vi "Vision Processing.vi"(4 "error in (no error)":errorcluster, 6 "CameraDevRef":T1) -> ()   [LabVIEW 2011]
uses:
  <vilib>/Rock Robotics/WPI/Camera/WPI_CameraDevRef.ctl
  Robot Global Data.vi
  <vilib>/vision/NI_Vision_Development_Module.lvlib
panel:
  in  "Scale":bool=TRUE
  out "Waveform Chart":dynamicdata(graph)
  out "Turret Movement Time":u32
  out "Target Identify Time":u32
  in  "Run Calculations":bool
  out "Raw Turret":dbl
  out "Target X Coord":dbl
  out "Target Distance":dbl
  out "Target Y Coord":dbl
  out "Distance Array":dbl[](array[numeric])
  in  "Scaler":dbl=0.85
  in  "Lower Speed Limit":dbl=0.05
  out "Number of Rectangles Visible":dbl
  out "Y Position Array":dbl[](array[numeric])
  out "X Position Array":dbl[](array[numeric])
  in  "View":bool
  out "Target Info":T2(array[cluster])
  in  "Area Size Limit":i32=444
  in  "Particle Count Limit":i32=8
  in  "Score Limits":T3={"Rect Coverage"=76.0, "Aspect Ratio"=40.0, "X Edge Strength"=40.0, "Y Edge Strength"=60.0}
  in  "Processing":enum32{"Color", "Intensity", "Intensity Open"}(tab)=enum."Intensity Open"
  in  "Luminance":i32=255
  in  "Saturation":i32=255
  in  "Hue":i32(knob)=65 scale=0.0..255.0
  in  "Margins":cluster{"Hue":i32, "Sat":i32, "Lum":i32}={"Hue"=20, "Sat"=27, "Lum"=30} {"Sat" scale=0.0..40.0; "Lum" scale=0.0..40.0; "Hue" scale=0.0..40.0}
  in  "Range":cluster{"Lower value":sgl, "Upper value":sgl}={"Lower value"=150.0, "Upper value"=255.0} {"Lower value" scale=0.0..255.0; "Upper value" scale=0.0..255.0}
  in  "Range":cluster{"Lower value":sgl, "Upper value":sgl}={"Lower value"=123.804344, "Upper value"=255.0} {"Lower value" scale=0.0..255.0; "Upper value" scale=0.0..255.0}
  in  "View":bool
  out "Processed Image":T4(plugin-control)
  out "Original Image":T4(plugin-control)
  # "Instructions:\nProcessing the reflective tape that is illuminated by a ring light can be based\non color or light intensity.\nParticles within the image are scored by rectangle coverage, aspect ratio, and\nfor being hollow with a bold edge. A particle is considered a target if all scores\nare above the score limits. Particles can be annotated -- surrounded by\na rectangle and scores drawn to the left .\nTo control the number of particles being scored, use the count limit and the size\nlimit."
  # "No Scale"
  # "To debug, Enable using the View button.\nFor color processing, you can click in the image to select the color for processing."
  # "Enable by clicking the View button.\nGreen scores are above the limit, orange are below. Inner/outer rect\nindicates all passed."
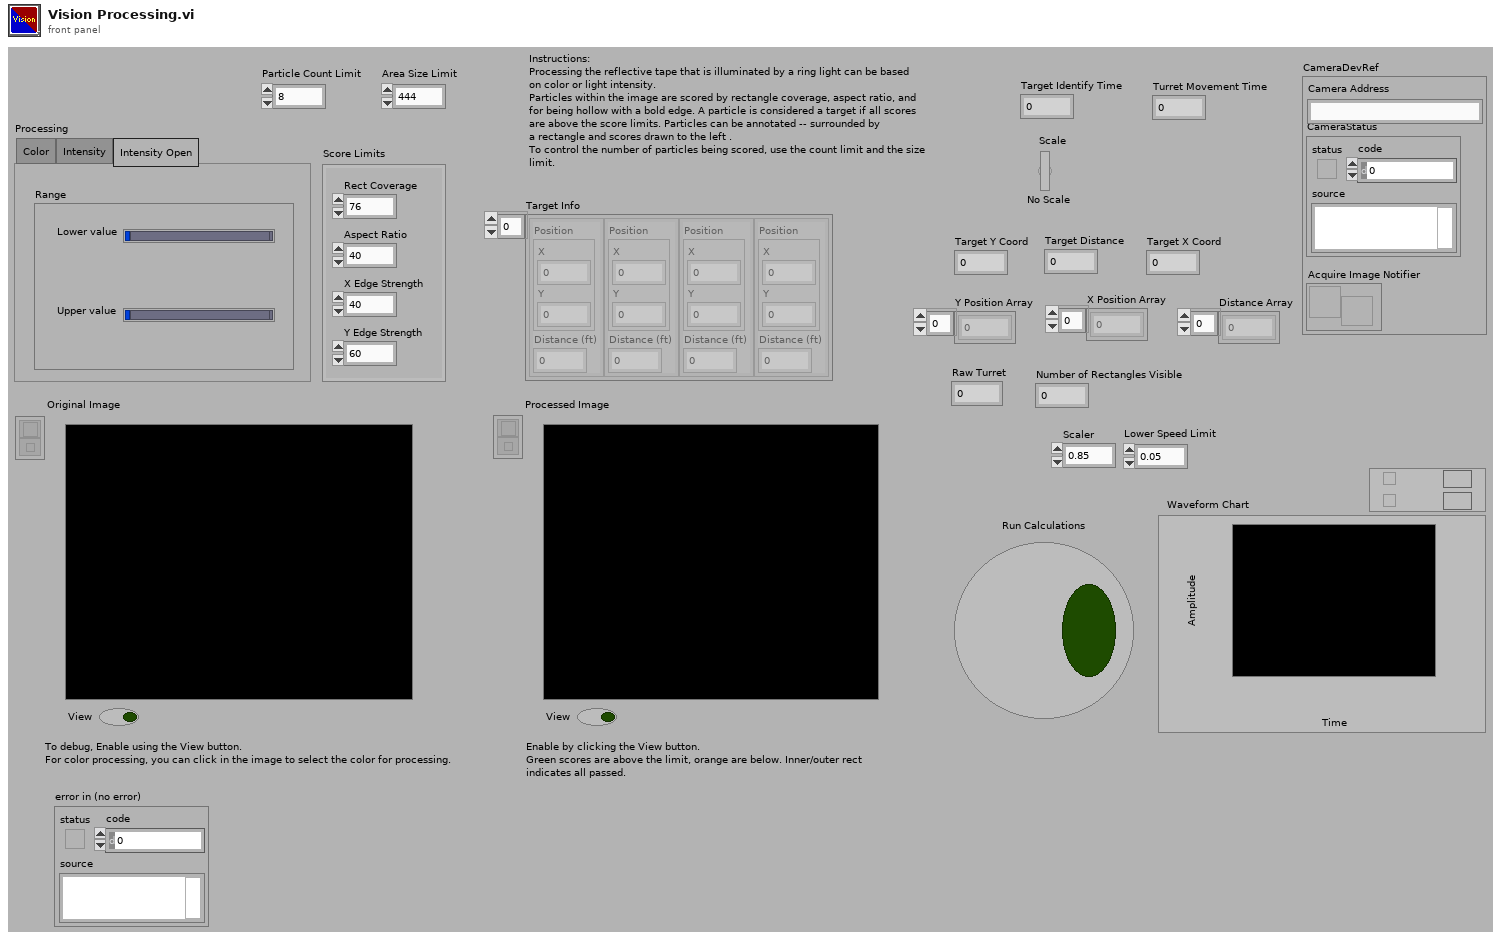
[diagram p1: front panel]
types:
  T1 = typedef "WPI_CameraDevRef.ctl" = cluster{"Camera Address":string, "CameraStatus":errorcluster, "Acquire Image Notifier":refnum<notifier>}
  T2 = cluster{"Position":cluster{"X":dbl, "Y":dbl}, "Distance (ft)":dbl}[]
  T3 = cluster{"Rect Coverage":dbl, "Aspect Ratio":dbl, "X Edge Strength":dbl, "Y Edge Strength":dbl}
  T4 = typedef "IMAQ Image.ctl" = refnum<image>
  T5 = typedef "Image Type" = u32
  T6 = enum32{"AutoM", "Close", "Dilate", "Erode", "Gradient", "Gradient out", "Gradient in", "Hit miss", "Open", "PClose", "POpen", "Thick", "Thin"}
  T7 = typedef "WPI_CameraImageSize.ctl" = enum16{"640x480", "320x240", "160x120"}
  T8 = cluster{"fps":i32, "compression":i32, "Image Size":T7}
  T9 = cluster{cluster{"Left":dbl, "Top":dbl, "Right":dbl, "Bottom":dbl}, dbl[]}[]
  T10 = cluster{"Left":dbl, "Top":dbl, "Right":dbl, "Bottom":dbl}
  T11 = cluster{"Target Center (-1 to 1)":cluster{"X":dbl, "Y":dbl}, "Distance (ft)":dbl}
  T12 = cluster{"Target Center (-1 to 1)":cluster{"X":dbl, "Y":dbl}, "Distance (ft)":dbl}[]
  T13 = typedef "WPI_JoystickDevRef.ctl" = cluster{"Device":T14}
  T14 = typedef "WPI_JoystickDeviceEnum.ctl" = enum16{"USB 1", "USB 2", "USB 3", "USB 4", "Kinect 1", "Kinect 2"}
  T15 = typedef "WPI_JoystickButtonState.ctl" = cluster{"Button 1":bool, "Button 2":bool, "Button 3":bool, "Button 4":bool, "Button 5":bool, "Button 6":bool, "Button 7":bool, "Button 8":bool, "Button 9":bool, "Button 10":bool, "Button 11":bool, "Button 12":bool}
  T16 = cluster{"axis 1 (x)":dbl, "axis 2 (y)":dbl, "axis 3 (throttle)":dbl, "axis 4":dbl, "axis 5":dbl, "axis 6":dbl}
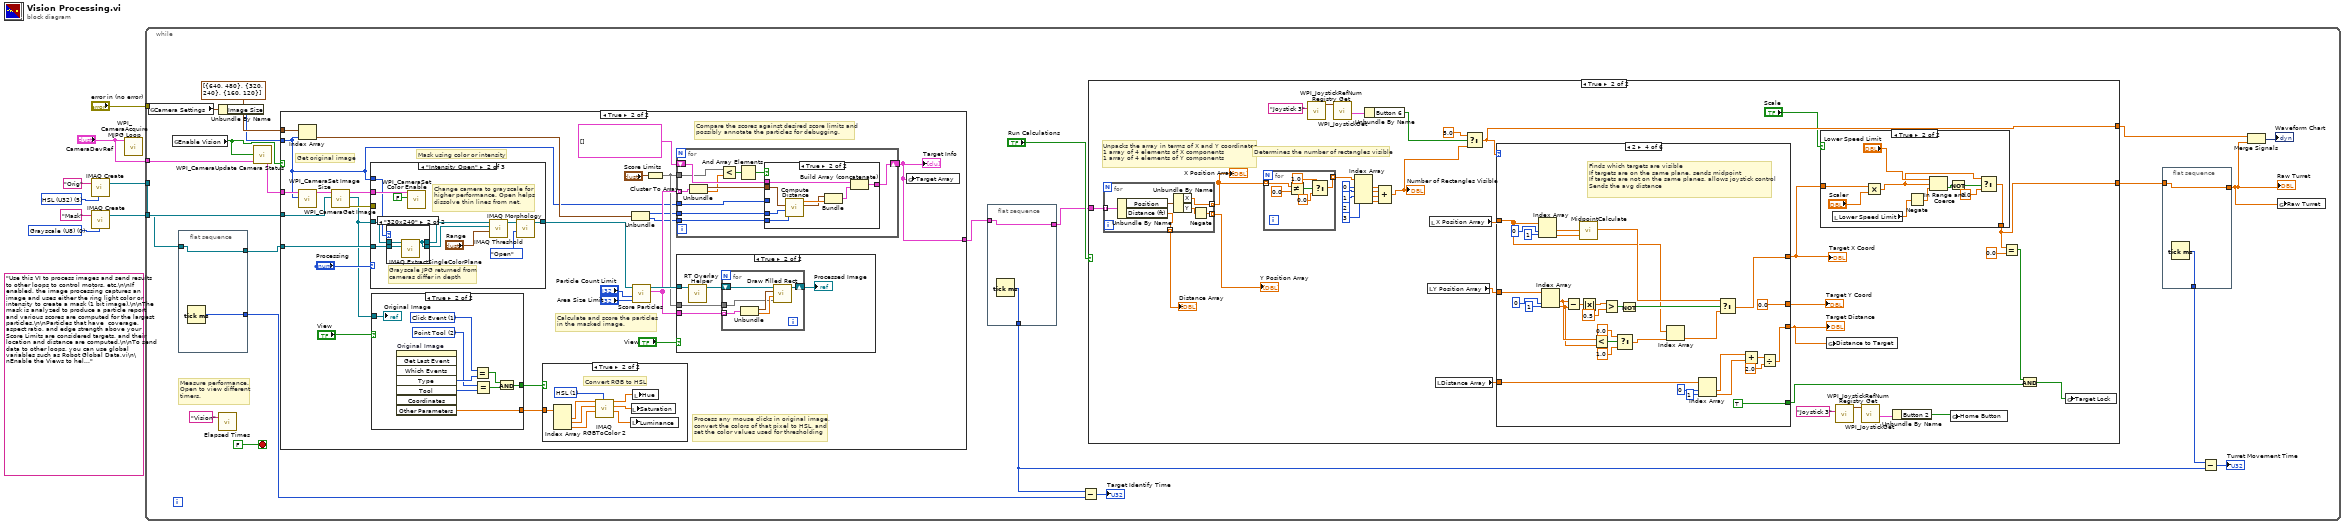
[diagram p0: block diagram]
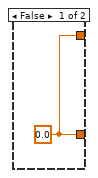
[diagram p2: hidden frame]
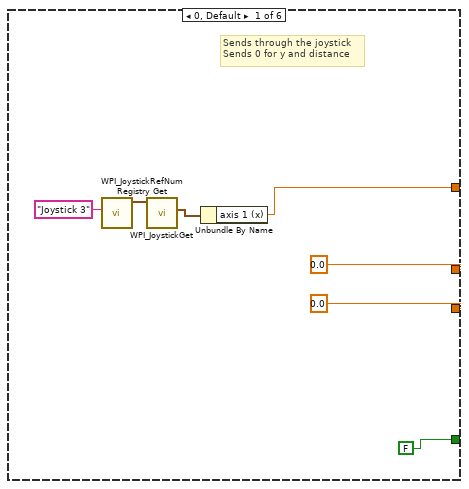
[diagram p4: hidden frame]
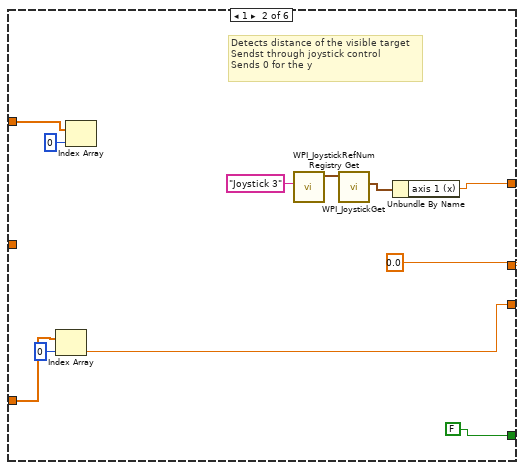
[diagram p5: hidden frame]
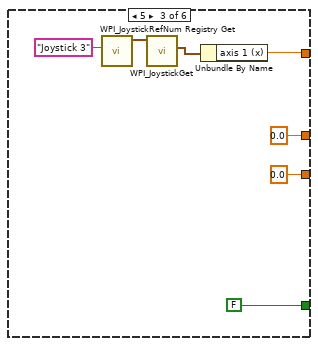
[diagram p6: hidden frame]
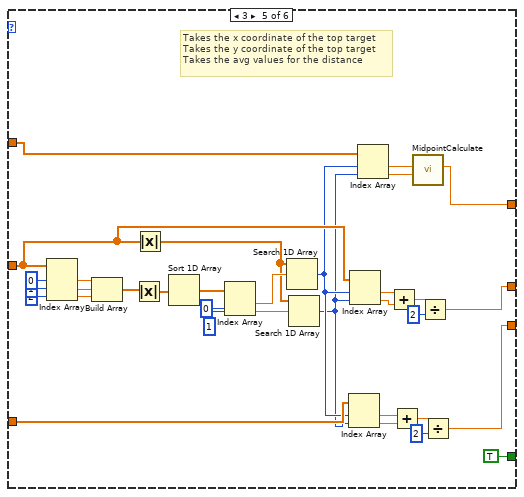
[diagram p7: hidden frame]
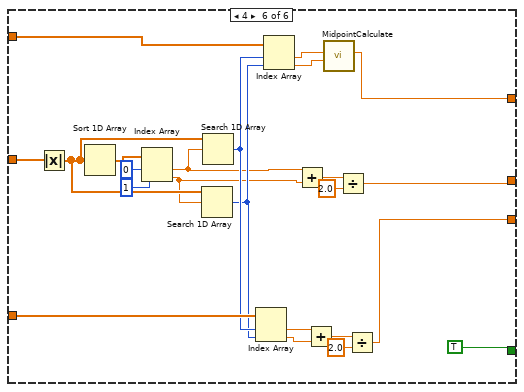
[diagram p8: hidden frame]
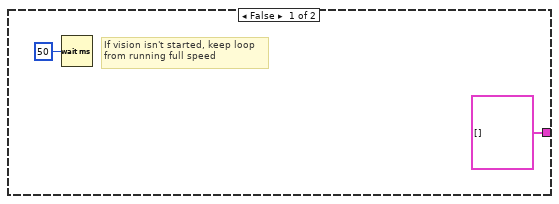
[diagram p9: hidden frame]
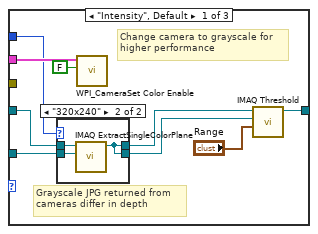
[diagram p11: hidden frame]
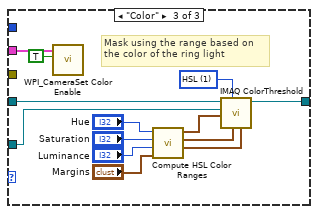
[diagram p14: hidden frame]
diagram:
  w3 = T5 0 items=["Grayscale (U8)", "Grayscale (I16)", "Grayscale (SGL)", "Complex (CSG)", "RGB (U32)", "HSL (U32)", "RGB (U64)", "Grayscale (U16)"] ("Image Type")
  (unwired) "Use this VI to process images and send results to other loops to control motors, etc.\n\nIf enabled, the image processing captures an image and uses either the ring light color or intensity to create a mask (1 bit image).\n\nThe mask is analyzed to produce a particle report and various scores are computed for the largest particles.\n\nParticles that have  coverage, aspect ratio, and edge strength above your Score Limits are considered targets, and their location and distance are computed.\n\nTo send data to other loops, you can use global variables such as Robot Global Data.vi\n\nEnable the Views to help debug color settings. Disable the View to speed up processing."
  w7 = T5 5 items=["Grayscale (U8)", "Grayscale (I16)", "Grayscale (SGL)", "Complex (CSG)", "RGB (U32)", "HSL (U32)", "RGB (U64)", "Grayscale (U16)"] ("Image Type")
  n1 = call "IMAQ Create"("Image Name"="Orig", "Image Type"=w7) -> ("New Image"=w6:T4)  [unwired: 2 in, 2 out]
  n2 = call "IMAQ Create"("Image Name"="Mask", "Image Type"=w3) -> ("New Image"=w1:T4)  [unwired: 2 in, 2 out]
  n3 = call <vilib>:"WPI_CameraAcquire MJPG Loop.vi"("CameraDevRef"="CameraDevRef") -> ()  [unwired: 11 in]
  n4 = while {
    tunnel: w6 -> [w30]
    tunnel: "CameraDevRef" -> [w29]
    tunnel: "error in (no error)" -> [_]
    tunnel: w1 -> [w20]
    stop <- FALSE stop-if-true
    # "Measure performance.\nOpen to view different\ntimers."
    n5 = global read "Robot Global Data.vi" "Camera Settings"() -> (w24:T8)
    n6 = global read "Robot Global Data.vi" "Enable Vision"() -> (w27:bool)
    n7 = flat-sequence {
      tunnel: [w37] -> w21
      tunnel: w20 -> [w37]
      tunnel: [w36] -> w16
      frame #0 {
        n8 = Tick Count (ms)() -> (millisecond timer value=w36:u32)
      }
    }
    n9 = Unbundle By Name(w24) -> ("Image Size"=w23:T7)
    n10 = call "Elapsed Times.vi"("Call Name"="Vision") -> ()  [unwired: 2 in, 1 out]
    n11 = call <vilib>:"WPI_CameraUpdate Camera Status.vi"("CameraDevRef In"=w29, "Enable Vision"=w27) -> ("CameraDevRef Out"=w28:T1)  [unwired: 3 in]
    n12 = case shown="True" w27 {
      tunnel: w30 -> [_ w229]
      tunnel: w28 -> [_ w225]
      tunnel: w21 -> [_ w216]
      tunnel: cluster{i32, i32}[] [{640, 480}, {320, 240}, {160, 120}] -> [_ w220]
      tunnel: w23 -> [_ w213]
      tunnel: [T2 [] w214] -> w19
      frame False {
        # "If vision isn't started, keep loop\nfrom running full speed"
        n13 = Wait (ms)(milliseconds to wait=u32 50) -> ()  [unwired: 1 out]
      }
      frame True {
        # "Compare the scores against desired score limits and\npossibly annotate the particles for debugging."
        # "Process any mouse clicks in original image,\nconvert the colors of that pixel to HSL, and\nset the color values used for thresholding"
        # "Calculate and score the particles\nin the masked image."
        # "Mask using color or intensity"
        # "Get original image"
        n14 = call <vilib>:"WPI_CameraSet Image Size.vi"("Image Size"=w213, "CameraDevRef"=w225) -> ("CameraDevRef Out"=w226:T1)  [unwired: 8 in, 1 out]
        n15 = Index Array(array=w220, index=w213) -> (element=w217:cluster{i32, i32})
        n16 = call <vilib>:"WPI_CameraGet Image.vi"("Image"=w229, "CameraDevRef"=w226) -> ("error out"=w227:errorcluster, "Image Out"=w215:T4, "CameraDevRef Out"=w228:T1)  [unwired: 7 in]
        n17 = case shown="\"Intensity Open\"" "Processing" {
          tunnel: w215 -> [w251 w263 w289]
          tunnel: [w254 w268 w288] -> w223
          tunnel: w228 -> [w252 w266 w279]
          tunnel: w227 -> [_ _ _]
          tunnel: w216 -> [w250 w264 w277]
          tunnel: w213 -> [w249 w265 _]
          frame "Intensity", Default {
            # "Grayscale JPG returned from\ncameras differ in depth"
            # "Change camera to grayscale for\nhigher performance"
            n18 = case shown="\"320x240\"" w249 {
              tunnel: w251 -> [w257 w260]
              tunnel: w250 -> [w256 w259]
              tunnel: [w257 w258] -> w248
              tunnel: [w256 w258] -> w247
              frame "640x480", Default {
              }
              frame "320x240" {
                n19 = call "IMAQ ExtractSingleColorPlane"("Image Dst"=w259, "Image Src"=w260) -> ("Image Dst Out"=w258:T4)  [unwired: 8 in, 1 out]
              }
            }
            n20 = call <vilib>:"WPI_CameraSet Color Enable.vi"("Color Enabled"=FALSE, "CameraDevRef"=w252) -> ()  [unwired: 8 in, 2 out]
            n21 = call "IMAQ Threshold"("Range"="Range", "Image Dst"=w247, "Image Src"=w248) -> ("Image Dst Out"=w254:T4)  [unwired: 3 in, 5 out]
          }
          frame "Intensity Open" {
            # "Grayscale JPG returned from\ncameras differ in depth"
            # "Change camera to grayscale for\nhigher performance. Open helps\ndissolve thin lines from net."
            n22 = case shown="\"320x240\"" w265 {
              tunnel: w263 -> [w273 w276]
              tunnel: w264 -> [w272 w275]
              tunnel: [w273 w274] -> w262
              tunnel: [w272 w274] -> w261
              frame "640x480", Default {
              }
              frame "320x240" {
                n23 = call "IMAQ ExtractSingleColorPlane"("Image Dst"=w275, "Image Src"=w276) -> ("Image Dst Out"=w274:T4)  [unwired: 8 in, 1 out]
              }
            }
            n24 = call <vilib>:"WPI_CameraSet Color Enable.vi"("Color Enabled"=FALSE, "CameraDevRef"=w266) -> ()  [unwired: 8 in, 2 out]
            n25 = call "IMAQ Threshold"("Range"="Range", "Image Dst"=w261, "Image Src"=w262) -> ("Image Dst Out"=w269:T4)  [unwired: 3 in, 5 out]
            n26 = call "IMAQ Morphology"("Operation"=T6."Open", "Image Src"=w269) -> ("Image Dst Out"=w268:T4)  [unwired: 8 in, 1 out]
          }
          frame "Color" {
            w287 = u16 1 items=["RGB", "HSL", "HSV", "HSI"] ("Color Mode")
            # "Mask using the range based on\nthe color of the ring light"
            n27 = call <vilib>:"WPI_CameraSet Color Enable.vi"("Color Enabled"=TRUE, "CameraDevRef"=w279) -> ()  [unwired: 8 in, 2 out]
            n28 = call "Compute HSL Color Ranges.vi"("Margins"="Margins", "Luminance"="Luminance", "Saturation"="Saturation", "Hue"="Hue") -> ("Lum Range"=w284:cluster{i32, i32}, "Sat Range"=w285:cluster{i32, i32}, "Hue Range"=w286:cluster{i32, i32})  [unwired: 5 in]
            n29 = call "IMAQ ColorThreshold"("Blue or Luma or Val or Inten Range"=w284, "Green or Sat Range"=w285, "Color Mode"=w287, "Red or Hue Range"=w286, "Image Dst"=w277, "Image Src"=w289) -> ("Image Dst Out"=w288:T4)  [unwired: 4 in, 1 out]
          }
        }
        n30 = case shown="True" "View" {
          tunnel: w215 -> [_ w309]
          tunnel: [_ w304] -> w222
          tunnel: [_ w301] -> w221
          frame False {
          }
          frame True {
            w302 = 2 items=["None", "Selection Tool", "Point Tool", "Line Tool", "Rectangle Tool", "Oval Tool", "Polygon Tool", "ClosedFreehandTool", "Annulus Tool", "Rotated Rectangle Tool", "Zoom Tool", "Pan Tool", "Polyline Tool", "Freehand Tool"] ("Tool")
            w303 = 1 items=["No Event"=0, "Click Event"=1, "Draw Event"=2, "Size Event"=4, "Scroll Event"=5, "Double Click Event"=8] ("Type")
            n31 = invoke on="Original Image" class="ImageControl" method="Get Last Event"() -> ("Type"=w305:i32, "Tool"=w308:i32, "Other Parameters"=w301:sgl[])  [unwired: 8 in, 5 out]
            n32 = Equal?(x=w303, y=w305) -> (x = y?=w306:bool)
            n33 = Equal?(x=w302, y=w308) -> (x = y?=w307:bool)
            n34 = And(x=w306, y=w307) -> (x .and. y?=w304:bool)
            "Original Image" <- w309
          }
        }
        n35 = case shown="True" w222 {
          tunnel: w221 -> [_ w246]
          frame False {
          }
          frame True {
            w245 = u16 1 items=["RGB", "HSL", "HSV", "HSI", "CIE L*a*b*", "CIE XYZ"] ("Color Mode")
            # "Convert RGB to HSL"
            n36 = Index Array(array=w246) -> (element #1=w244:sgl, element #2=w242:sgl, element #3=w240:sgl)  [unwired: 3 in]
            n37 = call "IMAQ RGBToColor 2"("Color Mode"=w245, "Blue value"=w240, "Green value"=w242, "Red value"=w244) -> ("Blue or Luma or Val or Inten or Z or b*value"=w239:dbl, "Green or Sat or Y or a* value"=w241:dbl, "Red or Hue or X or L* value"=w243:dbl)  [unwired: 4 in, 1 out]
            n38 = local write "Luminance"(w239) -> ()
            n39 = local write "Saturation"(w241) -> ()
            n40 = local write "Hue"(w243) -> ()
          }
        }
        n41 = Unbundle(w217) -> (w219:i32, w218:i32)
        n42 = call "Score Particles.vi"("Area Size Limit"="Area Size Limit", "Particle Count Limit"="Particle Count Limit", "Image Refnum in"=w223) -> ("Scored Particle Info"=w234:T9, "Image Refnum out"=w237:T4)  [unwired: 7 in]
        n43 = Cluster To Array(cluster="Score Limits") -> (array=w232:dbl[])
        n44 = for {
          shift-right: [w319] -> w214
          shift-left: T2 [] -> [w320]
          tunnel: w219 -> [w318]
          tunnel: w234 -> [w316] mode=indexing
          tunnel: w232 -> [w311]
          tunnel: w213 -> [w315]
          tunnel: w218 -> [w310]
          n45 = Unbundle(w316) -> (w317:T10, w312:dbl[])
          n46 = Less?(x=w311, y=w312) -> (x < y?=w314:bool[])
          n47 = And Array Elements(Boolean array=w314) -> (logical AND=w313:bool)
          n48 = case shown="True" w313 {
            tunnel: w320 -> [w321 w329]
            tunnel: [w321 w328] -> w319
            tunnel: w317 -> [_ w324]
            tunnel: w318 -> [_ w326]
            tunnel: w315 -> [_ _]
            tunnel: w310 -> [_ w323]
            frame False {
            }
            frame True {
              n49 = call "Compute Distance.vi"("Y Image Resolution"=w323, "X Image Resolution"=w326, "Bounding Box"=w324) -> ("Target Center (-1 to 1)"=w322:cluster{"X":dbl, "Y":dbl}, "Distance (ft)"=w325:dbl)  [unwired: 7 in]
              n50 = Bundle("Target Center (-1 to 1)"=w322, "Distance (ft)"=w325) -> (w327:T11)  [unwired: 1 in]
              n51 = Build Array (concatenate)(w329, w327) -> (w328:T12)
            }
          }
        }
        "Target Info" <- w214
        n52 = case shown="True" "View" {
          tunnel: w237 -> [_ w291]
          tunnel: w234 -> [_ w293]
          tunnel: w232 -> [_ w292]
          frame False {
          }
          frame True {
            n53 = call "RT Overlay Helper.vi"("Refnum in"=w291) -> ("Refnum out"=w294:T4)  [unwired: 10 in]
            n54 = for {
              shift-right: [w299] -> w290
              shift-left: w294 -> [w300]
              tunnel: w293 -> [w296] mode=indexing
              tunnel: w292 -> [w295]
              n55 = Unbundle(w296) -> (w297:T10, w298:dbl[])
              n56 = call "Draw Filled Rect.vi"("Limits"=w295, "Scores"=w298, "Bounding Box"=w297, "image in"=w300) -> ("image out"=w299:T4)  [unwired: 7 in]
            }
            "Processed Image" <- w290
          }
        }
        n57 = global write "Robot Global Data.vi" "Target Array"(w214) -> ()
      }
    }
    n58 = flat-sequence {
      tunnel: [w35] -> w18
      tunnel: w19 -> [w35]
      tunnel: [w34] -> w13
      frame #0 {
        n59 = Tick Count (ms)() -> (millisecond timer value=w34:u32)
      }
    }
    n60 = Subtract(x=w13, y=w16) -> (x-y=→"Target Identify Time":u32)
    n61 = case shown="True" "Run Calculations" {
      tunnel: w18 -> [_ w56]
      tunnel: [w38 w41] -> w17
      tunnel: [w38 w40] -> w10
      frame False {
        w38 = 0.0 ("f")
      }
      frame True {
        # "Determines the number of rectangles visible"
        # "Unpacks the array in terms of X and Y coordinates\n1 array of 4 elements of X components\n1 array of 4 elements of Y components"
        n62 = for {
          tunnel: [w208] -> w57 mode=indexing
          tunnel: [w209] -> w67 mode=indexing
          tunnel: w56 -> [w206] mode=indexing
          tunnel: [w205] -> w69 mode=indexing
          n63 = Unbundle By Name(w206) -> ("Position"=w210:cluster{"X":dbl, "Y":dbl}, "Distance (ft)"=w205:dbl)
          n64 = Unbundle By Name(w210) -> ("X"=w209:dbl, "Y"=w207:dbl)
          n65 = Negate(x=w207) -> (-x=w208:dbl)
        }
        "X Position Array" <- w67
        "Y Position Array" <- w57
        "Distance Array" <- w69
        n66 = for {
          tunnel: w67 -> [w90] mode=indexing
          tunnel: [w86] -> w66 mode=indexing
          n67 = Not Equal?(x=w90, y=0.0) -> (x != y?=w89:bool)
          n68 = Select(t=1.0, s=w89, f=0.0) -> (s? t:f=w86:dbl)
        }
        n69 = call <vilib>:"WPI_JoystickRefNum Registry Get.vi"("refnum name"="Joystick 3") -> ("JoystickDevRef"=w46:T13)  [unwired: 9 in, 1 out]
        n70 = call <vilib>:"WPI_JoystickGet.vi"("JoystickDevRef"=w46) -> ("Buttons"=w44:T15)  [unwired: 4 in, 2 out]
        n71 = Index Array(array=w66, index #1=0 ("index"), index #2=1 ("index"), index #3=2 ("index"), index #4=3 ("index")) -> (element #1=w64:dbl, element #2=w65:dbl, element #3=w63:dbl, element #4=w62:dbl)
        n72 = Unbundle By Name(w44) -> ("Button 6"=w43:bool)
        n73 = Compound Arithmetic op=ADD(w64, w65, w63, w62) -> (w55:dbl)
        "Number of Rectangles Visible" <- w55
        n74 = local read "Y Position Array"() -> (w72:dbl[])
        n75 = local read "X Position Array"() -> (w68:dbl[])
        n76 = local read "Distance Array"() -> (w73:dbl[])
        n77 = Select(t=5.0, s=w43, f=w55) -> (s? t:f=w40:dbl)
        n78 = case shown="2" w40 {
          tunnel: w68 -> [_ w104 _ w119 w165 w198]
          tunnel: [w92 w99 w110 w137 w162 w188] -> w71
          tunnel: [0.0 ("X") 0.0 ("X") 0.0 ("X") 0.0 ("X") w166 w187] -> w70
          tunnel: [0.0 ("X") w107 0.0 ("X") w130 w150 w182] -> w42
          tunnel: w72 -> [_ _ _ w146 w158 w203]
          tunnel: w73 -> [_ w109 _ w129 w153 w197]
          tunnel: [FALSE FALSE FALSE TRUE TRUE TRUE] -> w53
          frame 0, Default {
            # "Sends through the joystick\nSends 0 for y and distance"
            n79 = call <vilib>:"WPI_JoystickRefNum Registry Get.vi"("refnum name"="Joystick 3") -> ("JoystickDevRef"=w95:T13)  [unwired: 9 in, 1 out]
            n80 = call <vilib>:"WPI_JoystickGet.vi"("JoystickDevRef"=w95) -> ("Axes"=w93:T16)  [unwired: 4 in, 2 out]
            n81 = Unbundle By Name(w93) -> ("axis 1 (x)"=w92:dbl)
          }
          frame 1 {
            # "Detects distance of the visible target\nSendst through joystick control\nSends 0 for the y"
            n82 = Index Array(array=w109, index=0) -> (element=w107:dbl)
            n83 = Index Array(array=w104, index=0) -> ()  [unwired: 1 out]
            n84 = call <vilib>:"WPI_JoystickRefNum Registry Get.vi"("refnum name"="Joystick 3") -> ("JoystickDevRef"=w102:T13)  [unwired: 9 in, 1 out]
            n85 = call <vilib>:"WPI_JoystickGet.vi"("JoystickDevRef"=w102) -> ("Axes"=w100:T16)  [unwired: 4 in, 2 out]
            n86 = Unbundle By Name(w100) -> ("axis 1 (x)"=w99:dbl)
          }
          frame 5 {
            n87 = call <vilib>:"WPI_JoystickRefNum Registry Get.vi"("refnum name"="Joystick 3") -> ("JoystickDevRef"=w113:T13)  [unwired: 9 in, 1 out]
            n88 = call <vilib>:"WPI_JoystickGet.vi"("JoystickDevRef"=w113) -> ("Axes"=w111:T16)  [unwired: 4 in, 2 out]
            n89 = Unbundle By Name(w111) -> ("axis 1 (x)"=w110:dbl)
          }
          frame 2 {
            # "Finds which targets are visible\nIf targets are on the same plane, sends midpoint\nIf targets are not on the same planes, allows joystick control\nSends the avg distance"
            n90 = Index Array(array=w119, index #1=0 ("index"), index #2=1 ("index")) -> (element #1=w135:dbl, element #2=w134:dbl)
            n91 = Index Array(array=w146, index #1=0 ("index"), index #2=1 ("index")) -> (element #1=w125:dbl, element #2=w124:dbl)
            n92 = Subtract(x=w125, y=w124) -> (x-y=w143:dbl)
            n93 = call "MidpointCalculate.vi"("X2"=w134, "X1"=w135) -> ("Midpoint"=w138:dbl)  [unwired: 9 in]
            n94 = Absolute Value(x=w143) -> (abs(x)=w142:dbl)
            n95 = Less?(x=w125, y=w124) -> (x < y?=w123:bool)
            n96 = Greater?(x=w142, y=0.5) -> (0:w139:bool)
            n97 = Select(t=0.0, s=w123, f=1.0) -> (s? t:f=w120:dbl)
            n98 = Not(x=w139) -> (.not. x?=w140:bool)
            n99 = Index Array(array=w119, index=w120) -> (element=w118:dbl)
            n100 = Index Array(array=w129, index #1=0 ("index"), index #2=1 ("index")) -> (element #1=w128:dbl, element #2=w127:dbl)
            n101 = Select(t=w138, s=w140, f=w118) -> (s? t:f=w137:dbl)
            n102 = Add(x=w128, y=w127) -> (x+y=w133:dbl)
            n103 = Divide(x=w133, y=2.0) -> (x/y=w130:dbl)
          }
          frame 3 {
            # "Takes the x coordinate of the top target\nTakes the y coordinate of the top target\nTakes the avg values for the distance"
            n104 = Index Array(array=w158, index #1=0 ("index"), index #2=1 ("index"), index #3=2 ("index")) -> (element #1=w178:dbl, element #2=w177:dbl, element #3=w176:dbl)
            n105 = Build Array(w178, w177, w176) -> (w175:dbl[])
            n106 = Absolute Value(x=w175) -> (abs(x)=w169:dbl[])
            n107 = Absolute Value(x=w158) -> (abs(x)=w161:dbl[])
            n108 = Sort 1D Array(array=w169) -> (sorted array=w174:dbl[])
            n109 = Index Array(array=w174, index #1=0 ("index"), index #2=1 ("index")) -> (element #1=w170:dbl, element #2=w171:dbl)
            n110 = Search 1D Array(1D array=w161, element=w170) -> (index of element=w152:i32)  [unwired: 1 in]
            n111 = Search 1D Array(1D array=w161, element=w171) -> (index of element=w151:i32)  [unwired: 1 in]
            n112 = Index Array(array=w153, index #1=w152, index #2=w151) -> (element #1=w155:dbl, element #2=w154:dbl)
            n113 = Index Array(array=w158, index #1=w152, index #2=w151) -> (element #1=w160:dbl, element #2=w159:dbl)
            n114 = Index Array(array=w165, index #1=w152, index #2=w151) -> (element #1=w164:dbl, element #2=w163:dbl)
            n115 = Add(x=w160, y=w159) -> (x+y=w168:dbl)
            n116 = Add(x=w155, y=w154) -> (x+y=w156:dbl)
            n117 = call "MidpointCalculate.vi"("X2"=w163, "X1"=w164) -> ("Midpoint"=w162:dbl)  [unwired: 9 in]
            n118 = Divide(x=w168, y=2) -> (x/y=w166:dbl)
            n119 = Divide(x=w156, y=2) -> (x/y=w150:dbl)
          }
          frame 4 {
            n120 = Absolute Value(x=w203) -> (abs(x)=w199:dbl[])
            n121 = Sort 1D Array(array=w199) -> (sorted array=w202:dbl[])
            n122 = Index Array(array=w202, index #1=0 ("index"), index #2=1 ("index")) -> (element #1=w194:dbl, element #2=w193:dbl)
            n123 = Search 1D Array(1D array=w199, element=w193) -> (index of element=w195:i32)  [unwired: 1 in]
            n124 = Search 1D Array(1D array=w199, element=w194) -> (index of element=w196:i32)  [unwired: 1 in]
            n125 = Index Array(array=w197, index #1=w196, index #2=w195) -> (element #1=w184:dbl, element #2=w183:dbl)
            n126 = Index Array(array=w198, index #1=w196, index #2=w195) -> (element #1=w190:dbl, element #2=w189:dbl)
            n127 = Add(x=w194, y=w193) -> (x+y=w192:dbl)
            n128 = Add(x=w184, y=w183) -> (x+y=w185:dbl)
            n129 = call "MidpointCalculate.vi"("X2"=w189, "X1"=w190) -> ("Midpoint"=w188:dbl)  [unwired: 9 in]
            n130 = Divide(x=w192, y=2.0) -> (x/y=w187:dbl)
            n131 = Divide(x=w185, y=2.0) -> (x/y=w182:dbl)
          }
        }
        "Target Y Coord" <- w70
        "Target Distance" <- w42
        "Target X Coord" <- w71
        n132 = case shown="True" "Scale" {
          tunnel: w71 -> [w75 w84]
          tunnel: [w75 w76] -> w41
          frame False {
          }
          frame True {
            n133 = local read "Lower Speed Limit"() -> (w78:dbl)
            n134 = Multiply(x=w84, y="Scaler") -> (x*y=w83:dbl)
            n135 = Negate(x=w78) -> (-x=w79:dbl)
            n136 = In Range and Coerce(upper limit="Lower Speed Limit", x=w83, lower limit=w79) -> (In Range?=w80:bool)  [unwired: 1 out]
            n137 = Not(x=w80) -> (.not. x?=w81:bool)
            n138 = Select(t=w83, s=w81, f=0.0) -> (s? t:f=w76:dbl)
          }
        }
        n139 = global write "Robot Global Data.vi" "Distance to Target"(w42) -> ()
        n140 = call <vilib>:"WPI_JoystickRefNum Registry Get.vi"("refnum name"="Joystick 3") -> ("JoystickDevRef"=w50:T13)  [unwired: 9 in, 1 out]
        n141 = call <vilib>:"WPI_JoystickGet.vi"("JoystickDevRef"=w50) -> ("Buttons"=w48:T15)  [unwired: 4 in, 2 out]
        n142 = Unbundle By Name(w48) -> ("Button 2"=w47:bool)
        n143 = global write "Robot Global Data.vi" "Home Button"(w47) -> ()
        n144 = Equal?(x=w41, y=0.0) -> (x = y?=w52:bool)
        n145 = And(x=w52, y=w53) -> (x .and. y?=w51:bool)
        n146 = global write "Robot Global Data.vi" "Target Lock"(w51) -> ()
      }
    }
    n147 = flat-sequence {
      tunnel: [w33] -> w11
      tunnel: w17 -> [w33]
      tunnel: [w32] -> w14
      frame #0 {
        n148 = Tick Count (ms)() -> (millisecond timer value=w32:u32)
      }
    }
    n149 = Subtract(x=w14, y=w13) -> (x-y=→"Turret Movement Time":u32)
    n150 = Merge Signals(w10, w11) -> (→"Waveform Chart":dynamicdata)
    n151 = global write "Robot Global Data.vi" "Raw Turret"(w11) -> ()
    "Raw Turret" <- w11
  }
